vi "LoginCode.vi"() -> (0 "error out":errorcluster, 3 "Device Out":T1={"Name"="", "BaseURL"="", "AppKey"="", "Headers"=["Content-Type:application/json"], "Timeout"=10000})   [LabVIEW 2016]
uses:
  SkylineCluster.ctl
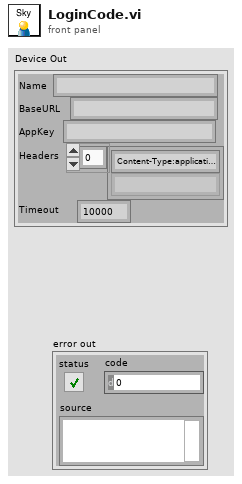
[diagram p1: front panel]
types:
  T1 = typedef "SkylineCluster.ctl" = cluster{"Name":string, "BaseURL":string, "AppKey":string, "Headers":string[], "Timeout":i32}
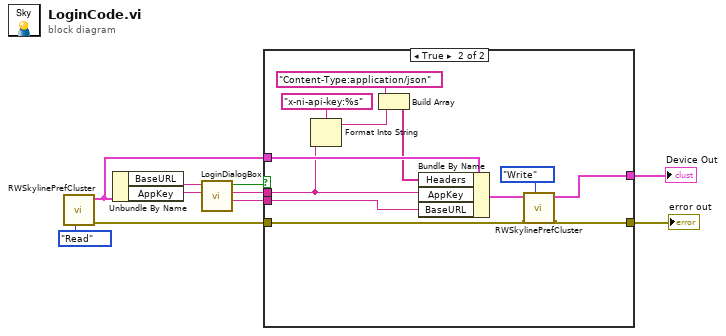
[diagram p0: block diagram]
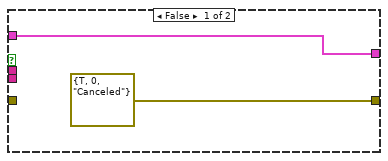
[diagram p2: hidden frame]
diagram:
  n1 = call "RWSkylinePrefCluster.vi"("Task"=enum16{"Read", "Write"}."Read") -> ("error out"=w1:errorcluster, "Device Out"=w4:T1)  [unwired: 9 in]
  n2 = Unbundle By Name(w4) -> ("BaseURL"=w3:string, "AppKey"=w6:string)
  n3 = call "LoginDialogBox.vi"("AppKey"=w6, "URL"=w3) -> ("URL out"=w2:string, "AppKey out"=w8:string, "OK?"=w7:bool)  [unwired: 7 in]
  n4 = case shown="True" w7 {
    tunnel: [errorcluster {"status"=TRUE, "code"=0, "source"="Canceled"} ("error out") w14] -> w10
    tunnel: w4 -> [w11 w24]
    tunnel: [w11 w16] -> w9
    tunnel: w8 -> [_ w22]
    tunnel: w1 -> [_ w15]
    tunnel: w2 -> [_ w13]
    frame False {
    }
    frame True {
      n5 = Format Into String(format string="x-ni-api-key:%s" ("Headers"), w22) -> (resulting string=w21:string)  [unwired: 2 in, 1 out]
      n6 = Build Array("Content-Type:application/json" ("Headers"), w21) -> (w19:string[])
      n7 = Bundle By Name(cluster=w24, "Headers"=w19, "AppKey"=w22, "BaseURL"=w13) -> (w18:T1)
      n8 = call "RWSkylinePrefCluster.vi"("Task"=enum16{"Read", "Write"}."Write", "error in (no error)"=w15, "Device In"=w18) -> ("error out"=w14:errorcluster, "Device Out"=w16:T1)  [unwired: 7 in]
    }
  }
  "Device Out" <- w9
  "error out" <- w10
